vi "Polymorphic.vi"   [LabVIEW 2017, in "G#MethodTemplates.lvclass"]
uses:
  <vilib>/addons/_AddQ/G#Templates/G#MethodTemplates/G#MethodTemplates.lvclass
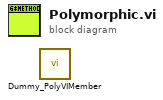
[diagram p0: block diagram]
diagram:
  n1 = call <vilib>:"Dummy_PolyVIMember.vi"() -> ()  [unwired: 20 in]
